vi "Camera.getBuffer.vi"(8 "error in (no error)":errorcluster, 10 "Get Image (-1: latest)":i32=-1, 11 "Camera.Simulated in":refnum<class "Camera.Simulated.lvclass">) -> (0 "error out":errorcluster, 2 "pixmap":u32[][](array[numeric]), 3 "Camera.Simulated out":refnum<class "Camera.Simulated.lvclass">)   [LabVIEW 2015, in "Camera.Simulated.lvclass"]
uses:
  Camera.Simulated.lvclass
  CircularBuffer/CircularBuffer.lvclass
  CircularBuffer.ImageData/CircularBuffer.ImageData.lvclass
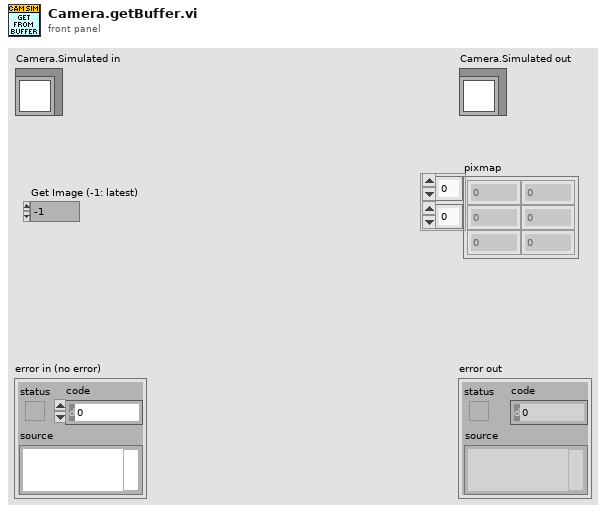
[diagram p1: front panel]
types:
  T1 = typedef "Camera.Simulated.lvclass/Dependencies--Cluster.ctl" = cluster{"CircularBuffer.ImageData":refnum<class "CircularBuffer.ImageData.lvclass">}
  T2 = typedef "imagedata.ctl" = cluster{"image type":i32, "image depth":i32, "image":u8[], "mask":u8[], "colors":u32[], "Rectangle":cluster{"left":i16, "top":i16, "right":i16, "bottom":i16}}
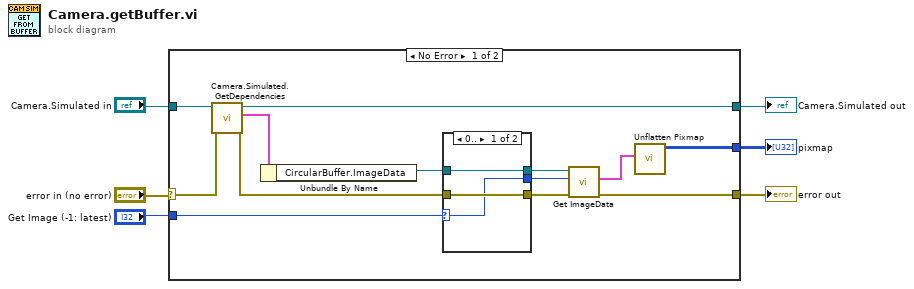
[diagram p0: block diagram]
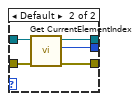
[diagram p2: hidden frame]
diagram:
  n1 = case shown="No Error" "error in (no error)" {
    selector: "error in (no error)" -> [w18 w29]
    tunnel: [w9 w29] -> w2
    tunnel: [w17 w28] -> w1
    tunnel: "Camera.Simulated in" -> [w19 w28]
    tunnel: "Get Image (-1: latest)" -> [w13 _]
    tunnel: [w7 _] -> w3
    frame No Error {
      n2 = call "Camera.Simulated.GetDependencies.vi"("error in (no error)"=w18, "Camera.Simulated"=w19) -> ("error out"=w14:errorcluster, "Dependencies"=w16:T1, "Camera.Simulated"=w17:refnum<class "Camera.Simulated.lvclass">)  [unwired: 7 in]
      n3 = Unbundle By Name(w16) -> ("CircularBuffer.ImageData"=w15:refnum<class "CircularBuffer.ImageData.lvclass">)
      n4 = case shown="0.." w13 {
        selector: w13 -> [w20 _]
        tunnel: w15 -> [w22 w27]
        tunnel: [w22 w26] -> w11
        tunnel: [w20 w25] -> w12
        tunnel: [w21 w24] -> w10
        tunnel: w14 -> [w21 w23]
        frame 0.. {
        }
        frame Default {
          n5 = call "Get CurrentElementIndex.vi"("error in (no error)"=w23, "CircularBuffer"=w27) -> ("error out"=w24:errorcluster, "Current Element index"=w25:i32, "CircularBuffer out"=w26:refnum<class "CircularBuffer.ImageData.lvclass">)  [unwired: 7 in]
        }
      }
      n6 = call "Get ImageData.vi"("error in (no error)"=w10, "GetElement (-1: Current)"=w12, "CircularBuffer.ImageData"=w11) -> ("error out"=w9:errorcluster, "ImageData"=w8:T2)  [unwired: 6 in, 1 out]
      n7 = call <vilib>:"Unflatten Pixmap.vi"("image data"=w8) -> ("24-bit pixmap"=w7:u32[][])  [unwired: 4 in, 6 out]
    }
    frame Error {
    }
  }
  "error out" <- w2
  "Camera.Simulated out" <- w1
  "pixmap" <- w3
